vi "Acquire.vi"(8 "error in (no error)":errorcluster, 9 "Data Queue":refnum<queue>, 10 "Data Notifier":refnum<notifier>, 11 "Hardware Resources in":T1={"DAQmx Channel 1"="", "DAQmx Channel 2"="", "DAQmx Channel 3"="", "DAQmx AI Task"="", "Channel 1 Name"="Battery Voltage", "Channel 2 Name"="Battery Current", "Channel 3 Name"="Brake torque", "Sample time"=50, "Samples per second"=1000.0, "Sample mode"=0, "Samples per channel"=0, "Offset Channel 1"=0.0, "Offset Channel 2"=0.0, "Offset Channel 3"=0.0, "Scale Channel 1"=0.0, "Scale Channel 2"=0.0, "Scale Channel 3"=0.0, "DAQmx Counter Channel"="", "Counter Name"="", "DAQmx Counter Task"=""} {"Sample mode" items=["Continuous Samples"=10123]}) -> (0 "error out":errorcluster, 3 "Hardware Resources out":T1={"DAQmx Channel 1"="", "DAQmx Channel 2"="", "DAQmx Channel 3"="", "DAQmx AI Task"="", "Channel 1 Name"="Battery Voltage", "Channel 2 Name"="Battery Current", "Channel 3 Name"="Brake torque", "Sample time"=50, "Samples per second"=1000.0, "Sample mode"=0, "Samples per channel"=0, "Offset Channel 1"=0.0, "Offset Channel 2"=0.0, "Offset Channel 3"=0.0, "Scale Channel 1"=0.0, "Scale Channel 2"=0.0, "Scale Channel 3"=0.0, "DAQmx Counter Channel"="", "Counter Name"="", "DAQmx Counter Task"=""} {"Sample mode" items=["Continuous Samples"=10123]})   [LabVIEW 2018, in "Acquisition.lvlib"]
doc: "Perform the acquisition. Replace the contents of this diagram with calls to acquisition hardware."
uses:
  Acquisition.lvlib
  Hardware Configuration.ctl
  <vilib>/DAQmx/read.llb/DAQmx Read (Counter U32 1Chan 1Samp).vi
  <vilib>/DAQmx/miscellaneous.llb/DAQmx Fill In Error Info.vi
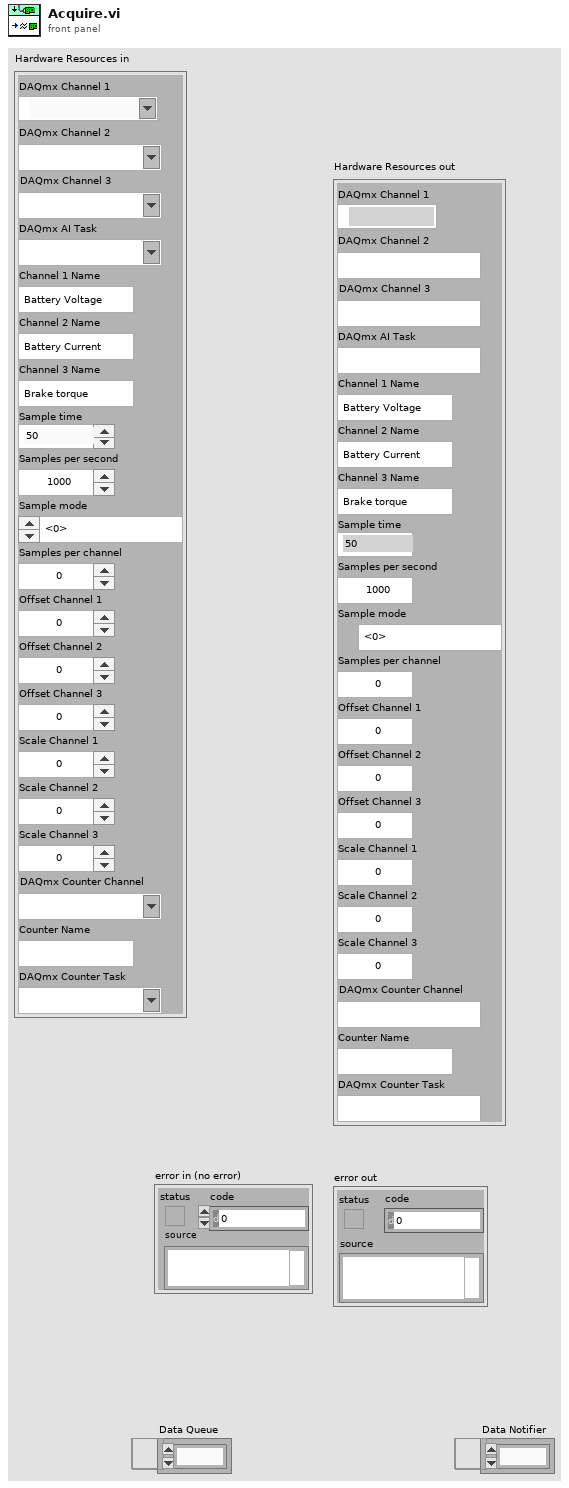
[diagram p1: front panel]
types:
  T1 = typedef "Acquisition.lvlib/Hardware Configuration.ctl" = cluster{"DAQmx Channel 1":tag, "DAQmx Channel 2":tag, "DAQmx Channel 3":tag, "DAQmx AI Task":refnum<k21>, "Channel 1 Name":string, "Channel 2 Name":string, "Channel 3 Name":string, "Sample time":u32, "Samples per second":dbl, "Sample mode":u16, "Samples per channel":i32, "Offset Channel 1":dbl, "Offset Channel 2":dbl, "Offset Channel 3":dbl, "Scale Channel 1":dbl, "Scale Channel 2":dbl, "Scale Channel 3":dbl, "DAQmx Counter Channel":tag, "Counter Name":string, "DAQmx Counter Task":refnum<k21>}
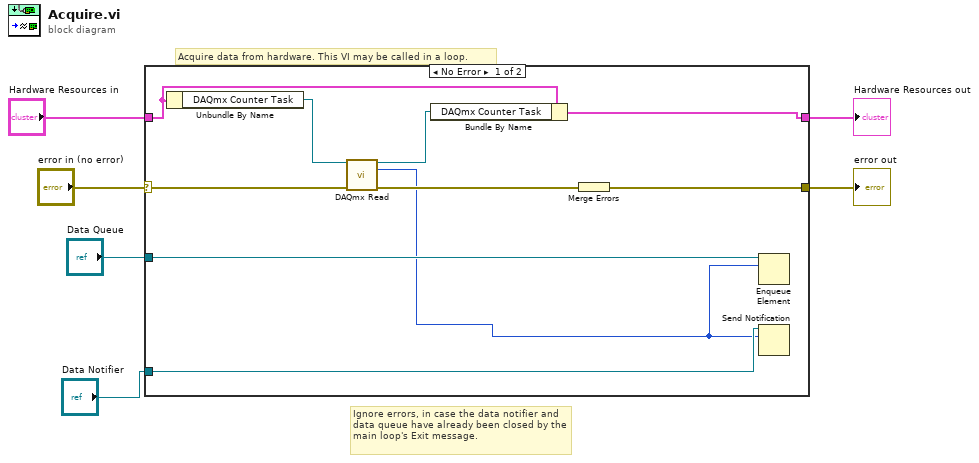
[diagram p0: block diagram]
diagram:
  # "Ignore errors, in case the data notifier and data queue have already been closed by the main loop's Exit message."
  # "Acquire data from hardware. This VI may be called in a loop."
  n1 = case shown="No Error" "error in (no error)" {
    selector: "error in (no error)" -> [w9 w17]
    tunnel: [w10 w17] -> w5
    tunnel: "Hardware Resources in" -> [w13 w18]
    tunnel: [w16 w18] -> w3
    tunnel: "Data Notifier" -> [w15 _]
    tunnel: "Data Queue" -> [w14 _]
    frame No Error {
      n2 = Unbundle By Name(w13) -> ("DAQmx Counter Task"=w12:refnum<k21>)
      n3 = call-poly <vilib>:"DAQmx Read.vi"("task/channels in"=w12, "error in"=w9) -> ("task out"=w8:refnum<k21>, "data"=w7:u32, "error out"=w11:errorcluster)  [unwired: 11 in]
      n4 = Bundle By Name(cluster=w13, "DAQmx Counter Task"=w8) -> (w16:T1)
      n5 = Merge Errors(w11) -> (w10:errorcluster)
      n6 = Enqueue Element(queue=w14, element=w7) -> ()  [unwired: 2 in, 3 out]
      n7 = Send Notification(notification=w7, notifier=w15) -> ()  [unwired: 1 in, 2 out]
    }
    frame Error {
    }
  }
  "Hardware Resources out" <- w3
  "error out" <- w5
